vi "Get Methods by Class Hierarchy.vi"(8 "error in (no error)":errorcluster, 11 "Class ID":string) -> (0 "error out":errorcluster, 3 "Methods by Class Hierarchy":T1(array[cluster]))   [LabVIEW 2023]
doc: "<b> </b> <b> </b>\n© 2017 Q Software Innovations, LLC\nwritten by Quentin \"Q\" Alldredge\nproduced in LabVIEW 2015\n\nsupport@qsoftwareinnovations.com\nwww.qsoftwareinnovations.com\n\nAll rights reserved.\n\nRedistribution and use in source and binary forms, with or without modification, are permitted provided that the following conditions are met:\n\n * Redistributions of source code must retain the above copyright notice, this list of conditions and the following disclaimer.\n * Redistributions in binary form must reproduce the above copyright notice, this list of conditions and the following disclaimer in the documentation and/or other materials provided with the distribution.\n * Neither the name of Q Software Innovations, LLC. nor the names of its contributors may be used to endorse or promote products derived from this software without specific prior written permission.\n\nTHIS SOFTWARE IS PROVIDED BY THE COPYRIGHT HOLDERS AND CONTRIBUTORS \"AS IS\" AND ANY EXPRESS OR IMPLIED WARRANTIES, INCLUDING, BUT NOT LIMITED TO, THE IMPLIED WARRANTIES OF MERCHANTABILITY AND FITNESS FOR A PARTICULAR PURPOSE ARE DISCLAIMED. IN NO EVENT SHALL THE COPYRIGHT OWNER OR CONTRIBUTORS BE LIABLE FOR ANY DIRECT, INDIRECT, INCIDENTAL, SPECIAL, EXEMPLARY, OR CONSEQUENTIAL DAMAGES (INCLUDING, BUT NOT LIMITED TO, PROCUREMENT OF SUBSTITUTE GOODS OR SERVICES; LOSS OF USE, DATA, OR PROFITS; OR BUSINESS INTERRUPTION) HOWEVER CAUSED AND ON ANY THEORY OF LIABILITY, WHETHER IN CONTRACT, STRICT LIABILITY, OR TORT (INCLUDING NEGLIGENCE OR OTHERWISE) ARISING IN ANY WAY OUT OF THE USE OF THIS SOFTWARE, EVEN IF ADVISED OF THE POSSIBILITY OF SUCH DAMAGE."
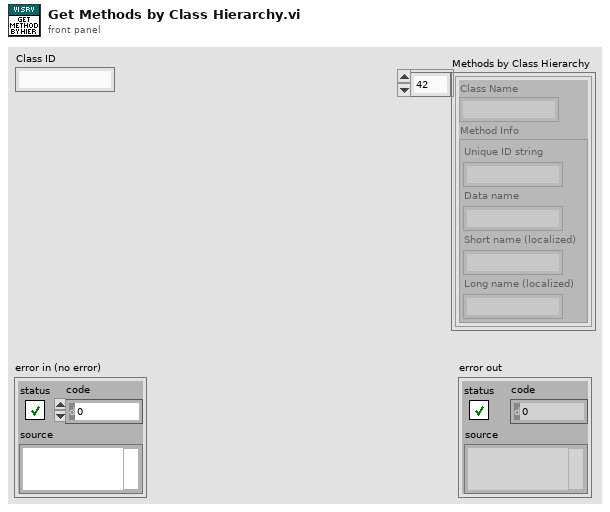
[diagram p1: front panel]
types:
  T1 = cluster{"Class Name":string, "Method Info":cluster{"Unique ID string":string, "Data name":string, "Short name (localized)":string, "Long name (localized)":string}}[]
  T2 = cluster{"Unique ID string":string, "Data name":string, "Short name (localized)":string, "Long name (localized)":string}[]
  T3 = cluster{"Unique ID string":string, "Parent ID string":string, "Class Name (unlocalized)":string, "Class Name (localized)":string}
  T4 = cluster{"Class Name (unlocalized)":string, "Property/Method Info":cluster{"Unique ID string":string, "Data name":string, "Short name (localized)":string, "Long name (localized)":string}}
  T5 = cluster{"Class Name (unlocalized)":string, "Property/Method Info":cluster{"Unique ID string":string, "Data name":string, "Short name (localized)":string, "Long name (localized)":string}}[]
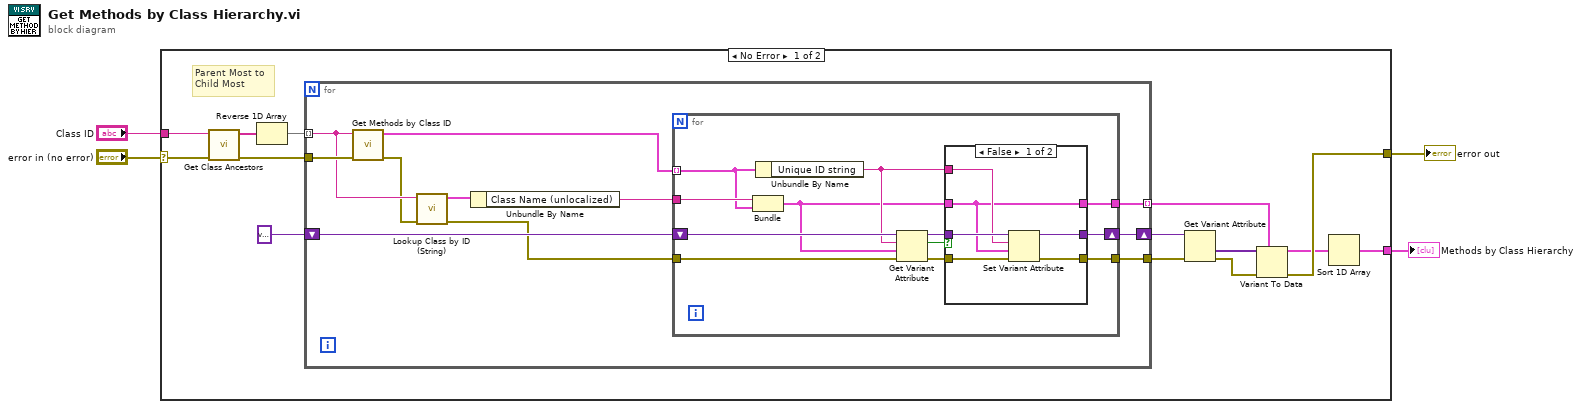
[diagram p0: block diagram]
diagram:
  n1 = case shown="No Error" "error in (no error)" {
    selector: "error in (no error)" -> [w18 w51]
    tunnel: [w7 w51] -> w3
    tunnel: "Class ID" -> [w17 _]
    tunnel: [w9 _] -> w1
    frame No Error {
      # "Parent Most to\nChild Most"
      n2 = call "Get Class Ancestors.vi"("error in (no error)"=w18, "Class ID"=w17) -> ("error out"=w16:errorcluster, "Class Ancestor IDs[]"=w15:string[])  [unwired: 8 in]
      n3 = Reverse 1D Array(array=w15) -> (reversed array=w14:string[])
      n4 = for {
        tunnel: w16 -> [w29]
        tunnel: w14 -> [w25] mode=indexing
        shift-right: [w27] -> w12
        shift-left: variant -> [w28]
        tunnel: [w20] -> w6 mode=indexing
        tunnel: [w19] -> w10
        n5 = call "Get Methods by Class ID.vi"("error in (no error)"=w29, "Class ID"=w25) -> ("error out"=w24:errorcluster, "Methods[]"=w26:T2)  [unwired: 8 in]
        n6 = call "Lookup Class by ID (String).vi"("error in (no error)"=w24, "Class ID"=w25) -> ("error out"=w23:errorcluster, "Class Information"=w22:T3)  [unwired: 7 in, 1 out]
        n7 = Unbundle By Name(w22) -> ("Class Name (unlocalized)"=w21:string)
        n8 = for {
          shift-right: [w38] -> w27
          shift-left: w28 -> [w41]
          tunnel: w26 -> [w33] mode=indexing
          tunnel: w23 -> [w40]
          tunnel: w21 -> [w34]
          tunnel: [w31] -> w20
          tunnel: [w30] -> w19
          n9 = Bundle("Class Name (unlocalized)"=w34, "Property/Method Info"=w33) -> (w32:T4)  [unwired: 1 in]
          n10 = Unbundle By Name(w33) -> ("Unique ID string"=w36:string)
          n11 = Get Variant Attribute(Variant=w41, name=w36, default value (empty Variant)=w32, error in=w40) -> (duplicate Variant=w37:variant, found=w39:bool, error out=w35:errorcluster)  [unwired: 1 out]
          n12 = case shown="False" w39 {
            tunnel: [w45 w50] -> w38
            tunnel: w37 -> [w47 w50]
            tunnel: w36 -> [w46 _]
            tunnel: w35 -> [w44 w48]
            tunnel: w32 -> [w43 w49]
            tunnel: [w43 w49] -> w31
            tunnel: [w42 w48] -> w30
            frame False {
              n13 = Set Variant Attribute(Variant=w47, name=w46, value=w43, error in=w44) -> (Variant out=w45:variant, error out=w42:errorcluster)  [unwired: 1 out]
            }
            frame True {
            }
          }
        }
      }
      n14 = Get Variant Attribute(Variant=w12, error in=w10) -> (values=w11:variant[], error out=w8:errorcluster)  [unwired: 2 in, 2 out]
      n15 = Variant To Data(error in=w8, type=w6, Variant=w11) -> (data=w5:T5, error out=w7:errorcluster)
      n16 = Sort 1D Array(array=w5) -> (sorted array=w9:T5)
    }
    frame Error {
    }
  }
  "error out" <- w3
  "Methods by Class Hierarchy" <- w1
